vi "Drive Status.vi"(9 "Disable\nDrive":bool, 10 "Enable\nDrive":bool, 11 "Motor":T1) -> (2 "Enabled?":bool, 3 "Drive Status":T2={"Status"=enum."Disabled", "Vsup Present"=FALSE, "Drive Fault"=FALSE, "Temp Fault"=FALSE})   [LabVIEW 2011]
uses:
  Controls/Drive Status.ctl
  <vilib>/LabVIEW Targets/FPGA/cRIO/cRIO-9505/controls.llb/_nicrio_cRIO-9505_DriveStatus.ctl
  Controls/Motor Names.ctl
  <vilib>/rvi/eio/common/nirviEmuTemplateMethod_errors.vi
  <vilib>/rvi/eio/common/nirviEmuTemplatePropertyGet_noerrors.vi
  <vilib>/eio/EIOMethodNode/EIOMethodNode.xnode
  <vilib>/eio/EIOPropertyNode/EIOPropertyNode.xnode
  <vilib>/rvi/eio/common/nirviEmuTemplatePropertyGet_errors.vi
  <vilib>/rvi/eio/common/nirviEmuTemplatePropertySet_errors.vi
  <vilib>/rvi/eio/common/nirviEmuTemplatePropertySet_noerrors.vi
panel:
  # "These status controls/indicators are used to enable/disable the drive and read fault information."
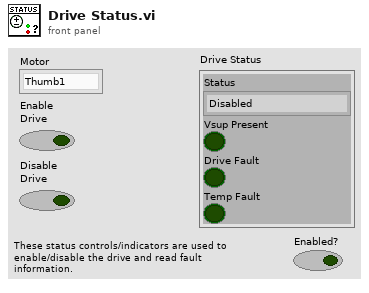
[diagram p1: front panel]
types:
  T1 = typedef "Motor Names.ctl" = enum16{"Thumb1", "Thumb2", "Thumb3", "Index1", "Index2", "Index3", "Redundant", "Middle1", "Middle2", "Middle3"}
  T2 = typedef "Drive Status.ctl" = cluster{"Status":T3, "Vsup Present":bool, "Drive Fault":bool, "Temp Fault":bool}
  T3 = typedef "_nicrio_cRIO-9505_DriveStatus.ctl" = enum8{"Enabled", "Disabled", "Disabled by Drive Fault", "Disabled by Temp. Fault", "Disabled by E-Stop", "Unknown"}
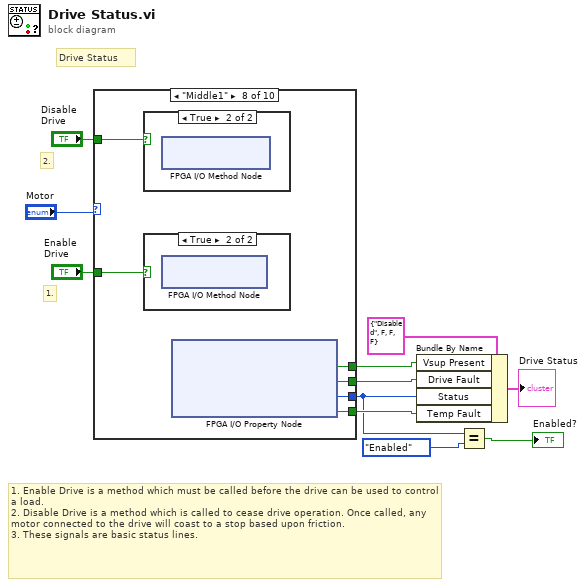
[diagram p0: block diagram]
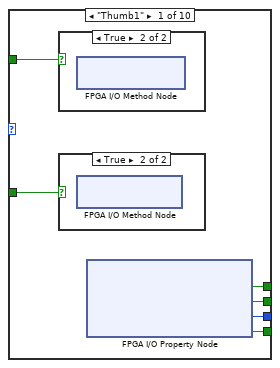
[diagram p2: hidden frame]
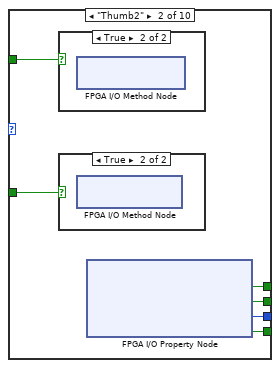
[diagram p5: hidden frame]
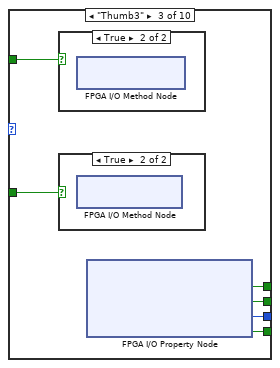
[diagram p8: hidden frame]
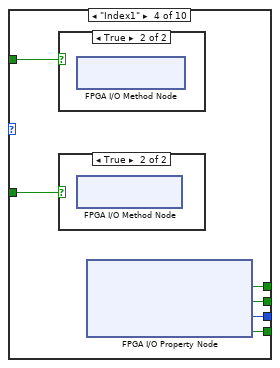
[diagram p11: hidden frame]
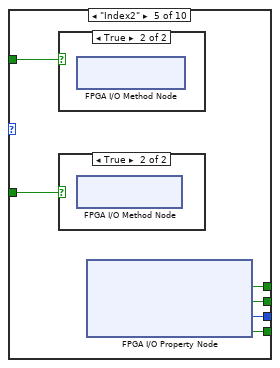
[diagram p14: hidden frame]
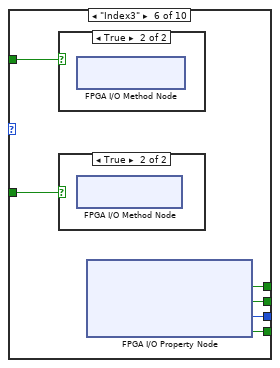
[diagram p17: hidden frame]
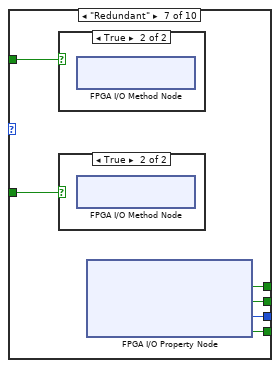
[diagram p20: hidden frame]
diagram:
  # "2."
  # "1."
  # "Drive Status"
  # "1. Enable Drive is a method which must be called before the drive can be used to control a load.\n2. Disable Drive is a method which is called to cease drive operation. Once called, any motor connected to the drive will coast to a stop based upon friction.\n3. These signals are basic status lines."
  n1 = case shown="\"Middle1\"" "Motor" {
    tunnel: "Enable\nDrive" -> [w16 w18 w24 w31 w36 w47 w48 w54 w60 w66]
    tunnel: "Disable\nDrive" -> [w17 w19 w25 w30 w37 w46 w49 w55 w61 w67]
    tunnel: [w15 w23 w29 w35 w41 w45 w53 w59 w65 w71] -> w7
    tunnel: [w14 w22 w28 w34 w40 w44 w52 w58 w64 w70] -> w6
    tunnel: [w12 w20 w26 w32 w38 w42 w50 w56 w62 w68] -> w5
    tunnel: [w13 w21 w27 w33 w39 w43 w51 w57 w63 w69] -> w2
    frame "Thumb1" {
      n2 = case shown="True" w17 {
        frame False {
        }
        frame True {
          n3 = xnode "FPGA I/O Method Node"() -> ()  [unwired: 1 in, 1 out]
        }
      }
      n4 = case shown="True" w16 {
        frame False {
        }
        frame True {
          n5 = xnode "FPGA I/O Method Node"() -> ()  [unwired: 1 in, 1 out]
        }
      }
      n6 = xnode "FPGA I/O Property Node"() -> ("Vsup Present"=w15:bool, "Drive Fault"=w14:bool, "Drive Status"=w13:T3, "Over Temperature Fault"=w12:bool)  [unwired: 1 in, 1 out]
    }
    frame "Thumb2" {
      n7 = case shown="True" w19 {
        frame False {
        }
        frame True {
          n8 = xnode "FPGA I/O Method Node"() -> ()  [unwired: 1 in, 1 out]
        }
      }
      n9 = case shown="True" w18 {
        frame False {
        }
        frame True {
          n10 = xnode "FPGA I/O Method Node"() -> ()  [unwired: 1 in, 1 out]
        }
      }
      n11 = xnode "FPGA I/O Property Node"() -> ("Vsup Present"=w23:bool, "Drive Fault"=w22:bool, "Drive Status"=w21:T3, "Over Temperature Fault"=w20:bool)  [unwired: 1 in, 1 out]
    }
    frame "Thumb3" {
      n12 = case shown="True" w25 {
        frame False {
        }
        frame True {
          n13 = xnode "FPGA I/O Method Node"() -> ()  [unwired: 1 in, 1 out]
        }
      }
      n14 = case shown="True" w24 {
        frame False {
        }
        frame True {
          n15 = xnode "FPGA I/O Method Node"() -> ()  [unwired: 1 in, 1 out]
        }
      }
      n16 = xnode "FPGA I/O Property Node"() -> ("Vsup Present"=w29:bool, "Drive Fault"=w28:bool, "Drive Status"=w27:T3, "Over Temperature Fault"=w26:bool)  [unwired: 1 in, 1 out]
    }
    frame "Index1" {
      n17 = case shown="True" w30 {
        frame False {
        }
        frame True {
          n18 = xnode "FPGA I/O Method Node"() -> ()  [unwired: 1 in, 1 out]
        }
      }
      n19 = case shown="True" w31 {
        frame False {
        }
        frame True {
          n20 = xnode "FPGA I/O Method Node"() -> ()  [unwired: 1 in, 1 out]
        }
      }
      n21 = xnode "FPGA I/O Property Node"() -> ("Vsup Present"=w35:bool, "Drive Fault"=w34:bool, "Drive Status"=w33:T3, "Over Temperature Fault"=w32:bool)  [unwired: 1 in, 1 out]
    }
    frame "Index2" {
      n22 = case shown="True" w37 {
        frame False {
        }
        frame True {
          n23 = xnode "FPGA I/O Method Node"() -> ()  [unwired: 1 in, 1 out]
        }
      }
      n24 = case shown="True" w36 {
        frame False {
        }
        frame True {
          n25 = xnode "FPGA I/O Method Node"() -> ()  [unwired: 1 in, 1 out]
        }
      }
      n26 = xnode "FPGA I/O Property Node"() -> ("Vsup Present"=w41:bool, "Drive Fault"=w40:bool, "Drive Status"=w39:T3, "Over Temperature Fault"=w38:bool)  [unwired: 1 in, 1 out]
    }
    frame "Index3" {
      n27 = case shown="True" w46 {
        frame False {
        }
        frame True {
          n28 = xnode "FPGA I/O Method Node"() -> ()  [unwired: 1 in, 1 out]
        }
      }
      n29 = case shown="True" w47 {
        frame False {
        }
        frame True {
          n30 = xnode "FPGA I/O Method Node"() -> ()  [unwired: 1 in, 1 out]
        }
      }
      n31 = xnode "FPGA I/O Property Node"() -> ("Vsup Present"=w45:bool, "Drive Fault"=w44:bool, "Drive Status"=w43:T3, "Over Temperature Fault"=w42:bool)  [unwired: 1 in, 1 out]
    }
    frame "Redundant" {
      n32 = case shown="True" w49 {
        frame False {
        }
        frame True {
          n33 = xnode "FPGA I/O Method Node"() -> ()  [unwired: 1 in, 1 out]
        }
      }
      n34 = case shown="True" w48 {
        frame False {
        }
        frame True {
          n35 = xnode "FPGA I/O Method Node"() -> ()  [unwired: 1 in, 1 out]
        }
      }
      n36 = xnode "FPGA I/O Property Node"() -> ("Vsup Present"=w53:bool, "Drive Fault"=w52:bool, "Drive Status"=w51:T3, "Over Temperature Fault"=w50:bool)  [unwired: 1 in, 1 out]
    }
    frame "Middle1" {
      n37 = case shown="True" w55 {
        frame False {
        }
        frame True {
          n38 = xnode "FPGA I/O Method Node"() -> ()  [unwired: 1 in, 1 out]
        }
      }
      n39 = case shown="True" w54 {
        frame False {
        }
        frame True {
          n40 = xnode "FPGA I/O Method Node"() -> ()  [unwired: 1 in, 1 out]
        }
      }
      n41 = xnode "FPGA I/O Property Node"() -> ("Vsup Present"=w59:bool, "Drive Fault"=w58:bool, "Drive Status"=w57:T3, "Over Temperature Fault"=w56:bool)  [unwired: 1 in, 1 out]
    }
    frame "Middle2" {
      n42 = case shown="True" w61 {
        frame False {
        }
        frame True {
          n43 = xnode "FPGA I/O Method Node"() -> ()  [unwired: 1 in, 1 out]
        }
      }
      n44 = case shown="True" w60 {
        frame False {
        }
        frame True {
          n45 = xnode "FPGA I/O Method Node"() -> ()  [unwired: 1 in, 1 out]
        }
      }
      n46 = xnode "FPGA I/O Property Node"() -> ("Vsup Present"=w65:bool, "Drive Fault"=w64:bool, "Drive Status"=w63:T3, "Over Temperature Fault"=w62:bool)  [unwired: 1 in, 1 out]
    }
    frame "Middle3" {
      n47 = case shown="True" w67 {
        frame False {
        }
        frame True {
          n48 = xnode "FPGA I/O Method Node"() -> ()  [unwired: 1 in, 1 out]
        }
      }
      n49 = case shown="True" w66 {
        frame False {
        }
        frame True {
          n50 = xnode "FPGA I/O Method Node"() -> ()  [unwired: 1 in, 1 out]
        }
      }
      n51 = xnode "FPGA I/O Property Node"() -> ("Vsup Present"=w71:bool, "Drive Fault"=w70:bool, "Drive Status"=w69:T3, "Over Temperature Fault"=w68:bool)  [unwired: 1 in, 1 out]
    }
  }
  n52 = Bundle By Name(cluster=T2 {"Status"=enum."Disabled", "Vsup Present"=FALSE, "Drive Fault"=FALSE, "Temp Fault"=FALSE} ("Drive Status"), "Vsup Present"=w7, "Drive Fault"=w6, "Status"=w2, "Temp Fault"=w5) -> (→"Drive Status":T2)
  n53 = Equal?(x=w2, y=_nicrio_cRIO-9505_DriveStatus."Enabled" ("Drive Status")) -> (x = y?=→"Enabled?":bool)
